vi "DataFinder_SearchText.vi"() -> ()   [LabVIEW 2023]
doc: "This example shows you how to use the DataFinder to quickly and easily search for descriptive information on measurement data. The example uses the \"Search Text\" VI to execute a text search and uses the \"Results To Waveforms\" VI to load and graphically display the mass data of the search results.\n\nRun the example, search with several search terms, and click the stop button to exit."
uses:
  <vilib>/userdefined/High Color/DFDataFinder.ctl
  <vilib>/DataFinder/Results to Waveforms (ddt).vi
  <vilib>/DataFinder/Close Reference (Results).vi
  <vilib>/DataFinder/Close Reference (DataFinder).vi
  <vilib>/userdefined/NI_DataFinder Controls.lvlib
  <vilib>/DataFinder/NI_DataFinder.lvlib
panel:
  in  "DataFinder":T1
  out "Result Signals":dynamicdata(graph)
  out "Results Count":i32 min=0 max=0
  in  "Search Text":string="Chris fail"
  out "Search Results":path[](array[path])
  in  "Search":bool
  in  "Stop Button":bool
  # "Overview: Searches for the given search text using a registered DataFinder and displays the resulting paths and signals.\nRequirements: Select a registered DataFinder which has indexed the TDM Server Demo Data.\nInstructions:\n1. Ensure that the selected DataFinder is already running.\n2. To use the predefined search values ensure the folder [all users]\\Documents\\National Instruments\\DataFinder or one of its parent folders is included in your search areas.\n3. Run the VI.\n4. Specify a value for Search Text and click the Search button.\n5. View the Search Results and Result Signals.\n6. Click Stop to stop the VI."
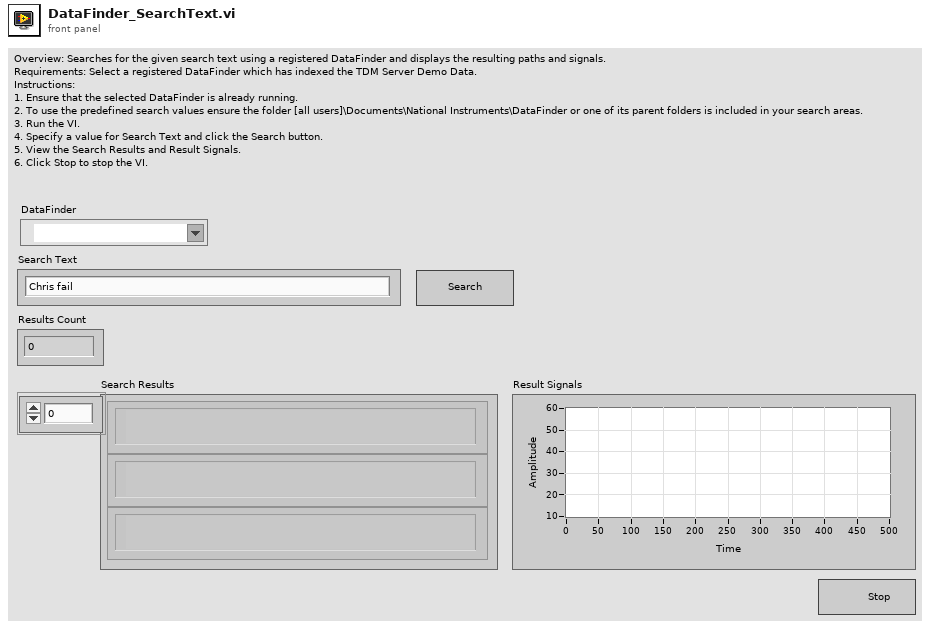
[diagram p1: front panel]
types:
  T1 = typedef "NI_DataFinder Controls.lvlib/DFDataFinder.ctl" = refnum<k21>
  T2 = typedef "NI_DataFinder Controls.lvlib/DFSearchResult.ctl" = refnum<k20>
  T3 = typedef "NI_DataFinder.lvlib/results elements.ctl" = cluster{"fullpaths":path[], "DataPlugin names":string[], "channel group names":string[], "channel names":string[]}
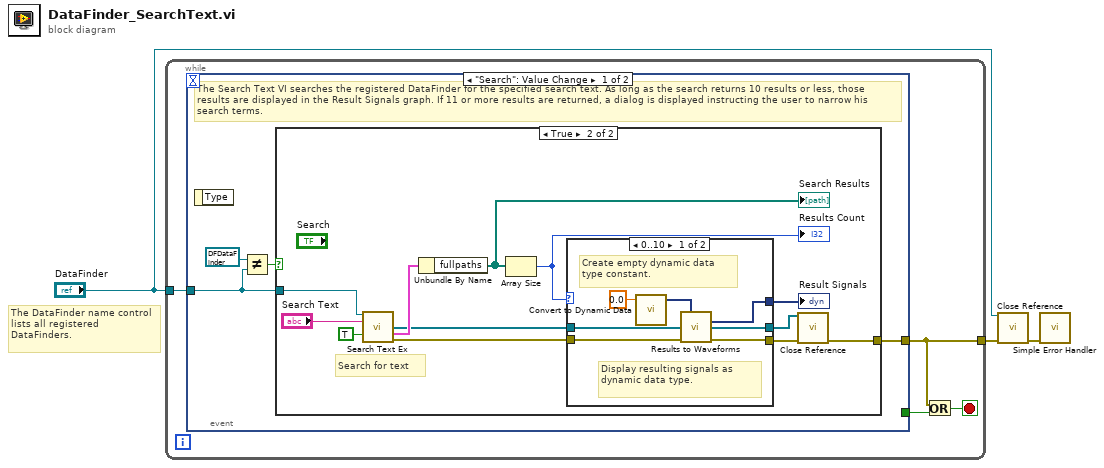
[diagram p0: block diagram]
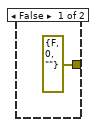
[diagram p2: hidden frame]
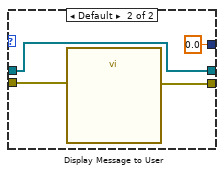
[diagram p3: hidden frame]
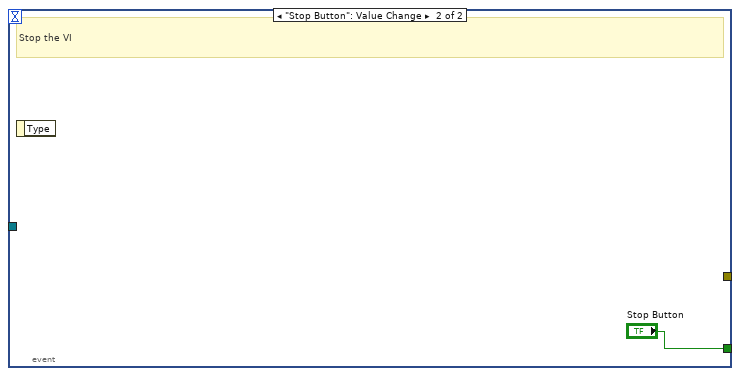
[diagram p4: hidden frame]
diagram:
  # "The DataFinder name control lists all registered DataFinders."
  n1 = while {
    tunnel: "DataFinder" -> [w7]
    tunnel: [w6] -> w1
    stop <- w4 stop-if-true
    n2 = event shown="[0] \"Search\": Value Change" {
      selector: _ -> [_ _]
      dyn-events: _ -> [_ _]
      timeout: _ -> [_ _]
      tunnel: [_ "Stop Button"] -> w5
      tunnel: w7 -> [w9 _]
      tunnel: [w11 _] -> w6
      event "Search": Value Change {
        # "The Search Text VI searches the registered DataFinder for the specified search text. As long as the search returns 10 results or less, those results are displayed in the Result Signals graph. If 11 or more results are returned, a dialog is displayed instructing the user to narrow his search terms."
        n3 = event-data() -> ()  [unwired: 1 in, 1 out]
        n4 = Not Equal?(x=T1 refnum ("DataFinder"), y=w9) -> (x != y?=w8:bool)
        n5 = case shown="True" w8 {
          tunnel: w9 -> [_ w22]
          tunnel: [errorcluster {"status"=FALSE, "code"=0, "source"=""} ("error out") w14] -> w11
          frame False {
          }
          frame True {
            # "Search for text"
            n6 = call <vilib>:"Search Text Ex.vi"("DataFinder reference"=w22, "search text"="Search Text", "fill results elements? (F)"=TRUE) -> ("result references out"=w19:T2[], "results elements"=w23:T3, "error out"=w21:errorcluster)  [unwired: 8 in, 2 out]
            n7 = Unbundle By Name(w23) -> ("fullpaths"=w20:path[])
            "Search Results" <- w20
            n8 = Array Size(array=w20) -> (size(s)=w18:i32)
            "Results Count" <- w18
            n9 = case shown="0..10" w18 {
              tunnel: w21 -> [w31 w35]
              tunnel: [w30 w34] -> w16
              tunnel: w19 -> [w29 w32]
              tunnel: [w26 0.0] -> w17
              tunnel: [w25 w32] -> w15
              frame 0..10 {
                # "Create empty dynamic data type constant."
                # "Display resulting signals as dynamic data type."
                n10 = call "Convert to Dynamic Data"("Double"=0.0) -> ("Dynamic Data Type"=w27:dynamicdata)  [unwired: 3 out]
                n11 = call-poly <vilib>:"Results to Waveforms.vi"("data type"=w27, "result references"=w29, "error in (no error)"=w31) -> ("signals out"=w26:dynamicdata, "result references out"=w25:T2[], "error out"=w30:errorcluster)  [unwired: 10 in]
              }
              frame Default {
                n12 = call "Display Message to User"("error in (no error)"=w35) -> ("error out"=w34:errorcluster)  [unwired: 2 in, 8 out]
              }
            }
            "Result Signals" <- w17
            n13 = call-poly <vilib>:"Close Reference.vi"("result references"=w15, "error in (no error)"=w16) -> ("error out"=w14:errorcluster)  [unwired: 13 in]
          }
        }
      }
      event "Stop Button": Value Change {
        # "Stop the VI"
        n14 = event-data() -> ()  [unwired: 1 in, 1 out]
      }
    }
    n15 = Or(x=w6, y=w5) -> (x .or. y?=w4:bool)
  }
  n16 = call-poly <vilib>:"Close Reference.vi"("DataFinder reference"="DataFinder", "error in (no error)"=w1) -> ("error out"=w3:errorcluster)  [unwired: 13 in]
  n17 = call <vilib>:"Simple Error Handler.vi"("error in (no error)"=w3) -> ()  [unwired: 4 in, 5 out]
